vi "Powershell Terminal.vi"(6 "command line":string="powershell.exe", 7 "Status":refnum<vi>, 8 "error in (no error)":errorcluster, 10 "working directory":path=path "c:/", 11 "StdIn":string="ping -n 3 127.0.0.1\nWrite-Host \"hello\"\nCopy-Item -Path \"C:\\intentionally\\invalid\\path\" -Destination \"C:\\another\\intentionally\\invalid\\path\"\nWrite-Error \"Another intentional error\"\nexit") -> (0 "error out":errorcluster, 1 "StdErr":string, 3 "StdOut":string)   [LabVIEW 2019]
uses:
  <vilib>/JKI/JKI DotNet System Exec/dotnet_system_exec/dotnet_system_exec.lvclass
  Build/Build.lvlib
panel:
  out "stdout":string
  out "stderr":string
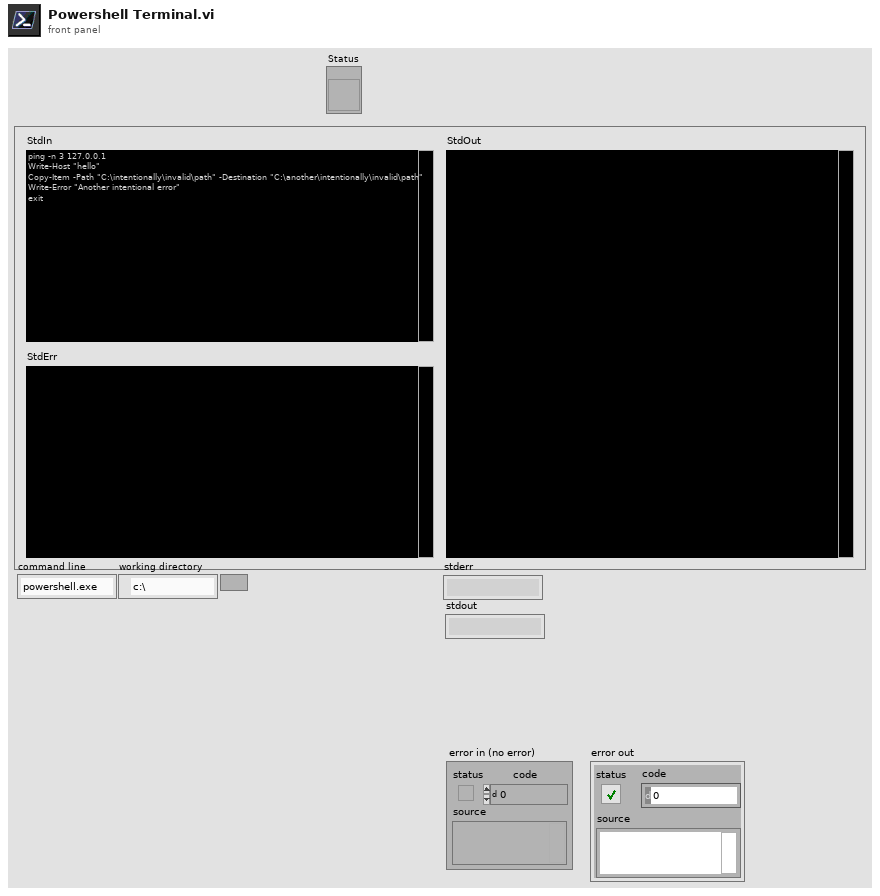
[diagram p1: front panel]
types:
  T1 = cluster{"stdout event":refnum<user-event>, "stderr event":refnum<user-event>, "process_exit event":refnum<user-event>}
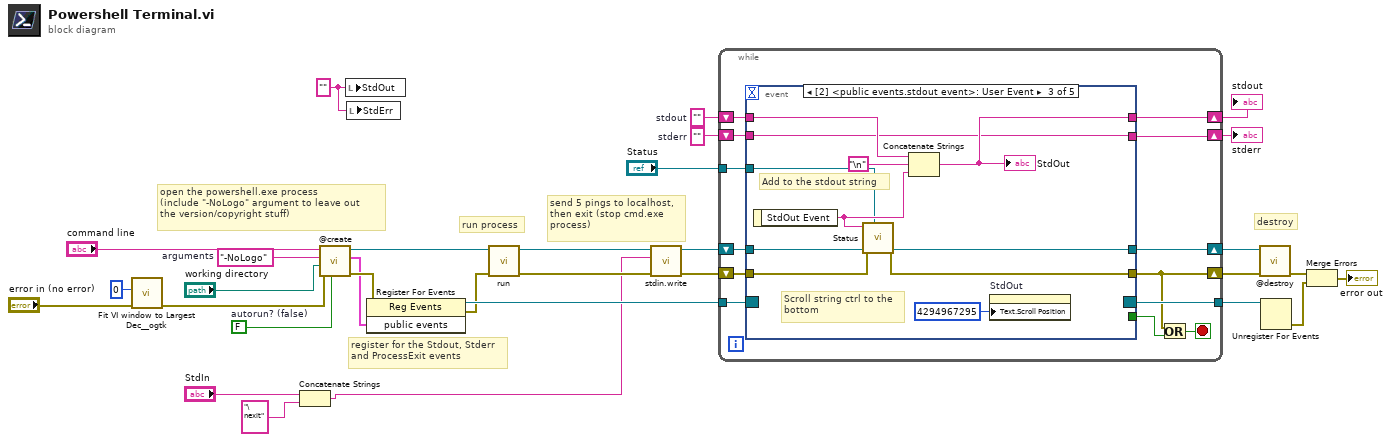
[diagram p0: block diagram]
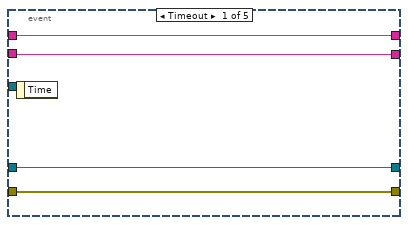
[diagram p2: hidden frame]
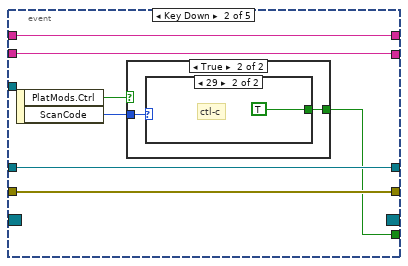
[diagram p3: hidden frame]
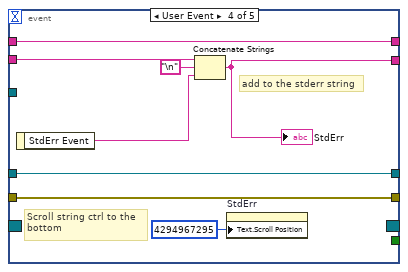
[diagram p6: hidden frame]
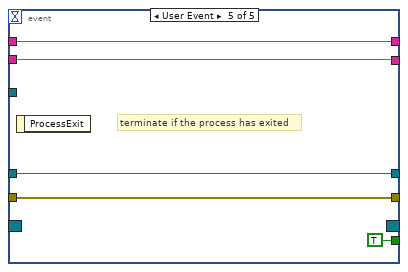
[diagram p7: hidden frame]
diagram:
  w16 = FALSE  # autorun? (false)
  w17 = "" ("Process File Name")
  w19 = ""  # stderr
  w7 = "-NoLogo"  # arguments
  w23 = ""  # stdout
  # "send 5 pings to localhost,\nthen exit (stop cmd.exe \nprocess)"
  # "destroy"
  # "register for the Stdout, Stderr \nand ProcessExit events"
  # "run process"
  # "open the powershell.exe process\n(include \"-NoLogo\" argument to leave out\nthe version/copyright stuff)"
  n1 = call <userlib>:"Fit VI window to Largest Dec__ogtk.vi"("error in (no error)"="error in (no error)", "border spacing (2 px)"=0) -> ("error out"=w11:errorcluster)  [unwired: 4 in, 1 out]
  n2 = Concatenate Strings("StdIn", "\nexit" ("string")) -> (w2:string)
  n3 = call <vilib>:"@create.vi"("autorun? (false)"=w16, "error in (no error)"=w11, "working directory (c:\\)"="working directory", "arguments (\"\")"=w7, "command line (cmd.exe)"="command line") -> ("error out"=w22:errorcluster, "public events"=w20:T1, "dotnet_system_exec out"=w30:refnum<class "dotnet_system_exec.lvclass">)  [unwired: 4 in]
  n4 = local write "StdOut"(w17) -> ()
  n5 = local write "StdErr"(w17) -> ()
  n6 = register-events(error in=w22, w20) -> (reference out=w29:refnum<event-registration>, error out=w21:errorcluster)  [unwired: 1 in]
  n7 = call <vilib>:"run.vi"("error in (no error)"=w21, "dotnet_system_exec in"=w30) -> ("error out"=w14:errorcluster, "dotnet_system_exec out"=w15:refnum<class "dotnet_system_exec.lvclass">)  [unwired: 8 in]
  n8 = call-dynamic "stdin.write.vi"("error in (no error)"=w14, "stdin"=w2, "dotnet_system_exec in"=w15) -> ("error out"=w12:errorcluster, "dotnet_system_exec out"=w13:refnum<class "dotnet_system_exec.lvclass">)  [unwired: 7 in]
  n9 = while {
    shift-right: [w44] -> w31
    shift-left: w13 -> [w43]
    shift-right: [w35] -> w27
    shift-left: w12 -> [w42]
    tunnel: w29 -> [w41]
    tunnel: [w40] -> w28
    shift-right: [w38] -> w5
    shift-left: w23 -> [w39]
    shift-right: [w36] -> w6
    shift-left: w19 -> [w37]
    tunnel: "Status" -> [w32]
    stop <- w34 stop-if-true
    n10 = event shown="[2] <public events.stdout event>: User Event" {
      selector: w41 -> [_ _ _ _ _]
      dyn-events: [_ _ _ _ _] -> w40
      timeout: _ -> [_ _ _ _ _]
      tunnel: [w48 w55 w68 w76 w79] -> w44
      tunnel: w43 -> [w48 w55 w68 w76 w79]
      tunnel: w42 -> [w47 w54 w59 w75 w78]
      tunnel: [w47 w54 w60 w75 w78] -> w35
      tunnel: w39 -> [w46 w53 w65 w72 w80]
      tunnel: [w46 w53 w66 w72 w80] -> w38
      tunnel: [_ w49 _ _ TRUE ("ProcessExit")] -> w33
      tunnel: w37 -> [w45 w52 w64 w73 w81]
      tunnel: [w45 w52 w64 w71 w81] -> w36
      tunnel: w32 -> [_ _ w61 _ _]
      event Timeout {
        n11 = event-data() -> ()  [unwired: 1 in, 1 out]
      }
      event Key Down {
        n12 = event-data() -> ("PlatMods.Ctrl"=w51:bool, "ScanCode"=w50:i16)  [unwired: 1 in]
        n13 = case shown="True" w51 {
          tunnel: w50 -> [_ w57]
          tunnel: [_ w56] -> w49
          frame False {
          }
          frame True {
            n14 = case shown="29" w57 {
              tunnel: [_ TRUE ("ProcessExit")] -> w56
              frame 0, Default {
              }
              frame 29 {
                # "ctl-c"
              }
            }
          }
        }
      }
      event User Event {
        # "Scroll string ctrl to the \nbottom"
        # "Add to the stdout string"
        n15 = event-data() -> ("StdOut Event"=w62:string)  [unwired: 1 in]
        n16 = call "Status.vi"("Reference"=w61, "error in (no error)"=w59, "Status"=w62) -> ("error out"=w60:errorcluster)  [unwired: 8 in]
        n17 = Concatenate Strings(w65, "\n", w62) -> (w66:string)
        "StdOut" <- w66
        n18 = property on="StdOut" class="Str"("Text.Scroll Position"=u32 4294967295) -> ()  [unwired: 2 in, 2 out]
      }
      event User Event {
        # "Scroll string ctrl to the \nbottom"
        # "add to the stderr string"
        n19 = event-data() -> ("StdErr Event"=w69:string)  [unwired: 1 in]
        n20 = Concatenate Strings(w73, "\n", w69) -> (w71:string)
        "StdErr" <- w71
        n21 = property on="StdErr" class="Str"("Text.Scroll Position"=u32 4294967295) -> ()  [unwired: 2 in, 2 out]
      }
      event User Event {
        # "terminate if the process has exited"
        n22 = event-data() -> ()  [unwired: 1 in, 1 out]
      }
    }
    n23 = Or(x=w35, y=w33) -> (x .or. y?=w34:bool)
  }
  "stderr" <- w6
  "stdout" <- w5
  n24 = call-dynamic "@destroy.vi"("error in (no error)"=w27, "dotnet_system_exec in"=w31) -> ("error out"=w26:errorcluster)  [unwired: 8 in, 1 out]
  n25 = Unregister For Events(event registration refnum=w28) -> (error out=w25:errorcluster)  [unwired: 1 in]
  n26 = Merge Errors(w26, w25) -> (→"error out":errorcluster)
